vi "RetryFileError.vi"(8 "error in (no error)":errorcluster, 10 "Path in":path, 11 "Path Array in":path[](array[path])) -> (0 "error out":errorcluster, 3 "Path Array out":path[](array[path]), 6 "Retry":bool)   [LabVIEW 2014]
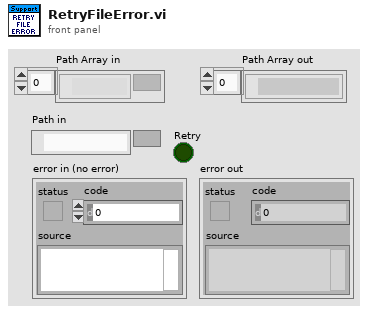
[diagram p1: front panel]
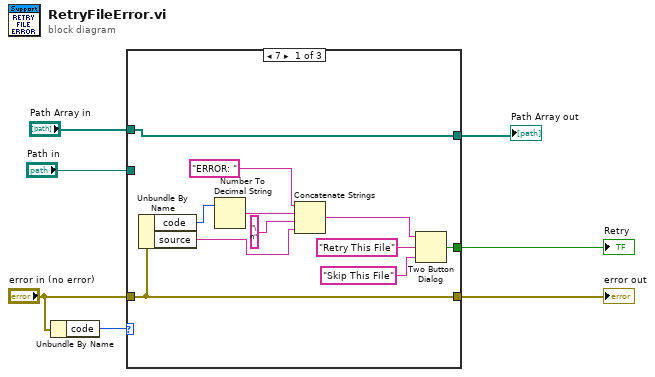
[diagram p0: block diagram]
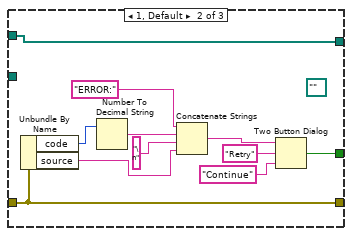
[diagram p2: hidden frame]
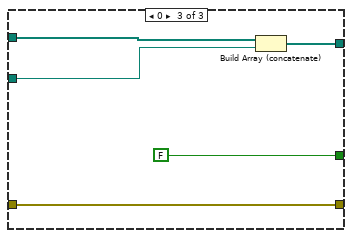
[diagram p3: hidden frame]
diagram:
  n1 = Unbundle By Name("error in (no error)") -> ("code"=w6:i32)
  n2 = case shown="7" w6 {
    tunnel: [w9 w27 w34] -> w7
    tunnel: "error in (no error)" -> [w9 w27 w34]
    tunnel: [w16 w25 FALSE ("T button?")] -> w4
    tunnel: "Path in" -> [_ _ w30]
    tunnel: "Path Array in" -> [w8 w19 w31]
    tunnel: [w8 w19 w32] -> w1
    frame 7 {
      n3 = Unbundle By Name(w9) -> ("code"=w14:i32, "source"=w11:string)
      n4 = Number To Decimal String(number=w14) -> (decimal integer string=w13:string)  [unwired: 1 in]
      n5 = Concatenate Strings("ERROR: ", w13, "\n" ("string"), w11) -> (w10:string)
      n6 = Two Button Dialog(message=w10, 1:"Skip This File" ("F button name (\"Cancel\")"), 2:"Retry This File" ("T button name (\"OK\")")) -> (T button?=w16:bool)
    }
    frame 1, Default {
      (unwired) path "" ("Path in")
      n7 = Unbundle By Name(w27) -> ("code"=w23:i32, "source"=w20:string)
      n8 = Number To Decimal String(number=w23) -> (decimal integer string=w22:string)  [unwired: 1 in]
      n9 = Concatenate Strings("ERROR:", w22, "\n" ("string"), w20) -> (w26:string)
      n10 = Two Button Dialog(message=w26, 1:"Continue" ("F button name (\"Cancel\")"), 2:"Retry" ("T button name (\"OK\")")) -> (T button?=w25:bool)
    }
    frame 0 {
      n11 = Build Array (concatenate)(w31, w30) -> (w32:path[])
    }
  }
  "error out" <- w7
  "Retry" <- w4
  "Path Array out" <- w1
